vi "Shooter logic.vi"(0 "Low Pressure?":bool, 1 "Fire Main":bool, 2 "Fire 3":bool, 3 "Fire 2":bool, 4 "Change Arm State":bool, 5 "Grabber Override":bool, 6 "Release to Retract":u32=750, 7 "Grabber Button":bool, 8 "Time Between Open and Shoot":u32=250) -> ()   [LabVIEW 2013]
uses:
  <vilib>/Rock Robotics/WPI/Solenoid/WPI_SolenoidValue.ctl
  <vilib>/Rock Robotics/WPI/Solenoid/WPI_SolenoidSetEnum.vi
  <vilib>/addons/control/pid/pid.llb/PID (DBL).vi
  Robot Global Data.vi
  <vilib>/addons/control/pid/NI_PID_pid.lvlib
panel:
  in  "Up Position":dbl format="%.2f"
  in  "Arms IN/OUT":enum16{"Out", "In"}(ring)
  in  "Grabber Override State":enum16{"Sensors", "Buttons"}(ring)
  in  "Grab Sweet Spot inches fron sensor":dbl
  out "PID reinitalize?":bool
  in  "Down Position":dbl format="%.2f"
  in  "PID gains":T1={"proportional gain (Kc)"=1.0, "integral time (Ti, min)"=0.01, "derivative time (Td, min)"=0.0} {"derivative time (Td, min)" format="%.3f"; "integral time (Ti, min)" format="%.3f"; "proportional gain (Kc)" format="%.3f"}
  out "Arms Position":T2
  in  "Grabber State":enum16{"Up", "Going Down", "Down", "Going Up"}(ring)
  out "Shooter Position":T2
  in  "Launcher State":T3(ring)
  out "Tick":u32
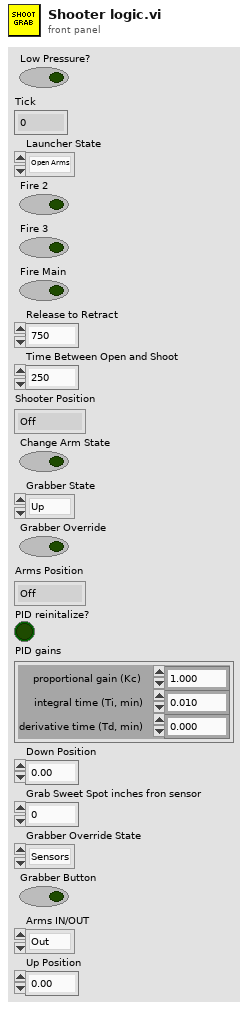
[diagram p1: front panel]
types:
  T1 = cluster{"proportional gain (Kc)":dbl, "integral time (Ti, min)":dbl, "derivative time (Td, min)":dbl}
  T2 = typedef "WPI_SolenoidValue.ctl" = enum16{"Off", "On", "Forward", "Reverse"}
  T3 = enum16{"Open Arms", "Arms Open", "Shoot", "Out", "Retract"}
  T4 = typedef "WPI_SolenoidDevRef.ctl" = cluster{"DevStatus":errorcluster, "Solenoid Module":T5, "Forward Solenoid Channel":T6, "Reverse Solenoid Channel":T6}
  T5 = typedef "FPGA_TypedefSolenoidModule.ctl" = enum16{"Solenoid Module 1", "Solenoid Module 2"}
  T6 = typedef "WPI_SolenoidChannel.ctl" = enum8{"Solenoid 1", "Solenoid 2", "Solenoid 3", "Solenoid 4", "Solenoid 5", "Solenoid 6", "Solenoid 7", "Solenoid 8", "Invalid"}
  T7 = typedef "WPI_DigitalInputDevRef.ctl" = cluster{"DevStatus":errorcluster, "DIO Channel":T8, "Digital Module":T9}
  T8 = typedef "FPGA_DIOChannel.ctl" = enum8{"DIO 1", "DIO 2", "DIO 3", "DIO 4", "DIO 5", "DIO 6", "DIO 7", "DIO 8", "DIO 9", "DIO 10", "DIO 11", "DIO 12", "DIO 13", "DIO 14", "Invalid"}
  T9 = typedef "FPGA_TypedefDigitalModule.ctl" = enum16{"Digital Module 1", "Digital Module 2"}
  T10 = typedef "WPI_AnalogChannelDevRef.ctl" = cluster{"DevStatus":errorcluster, "Analog Module":T11, "Analog Channel":T12}
  T11 = typedef "FPGA_TypedefAnalogModule.ctl" = enum16{"Analog Module 1", "Analog Module 2"}
  T12 = typedef "FPGA_AIChannel.ctl" = enum8{"AI 1", "AI 2", "AI 3", "AI 4", "AI 5", "AI 6", "AI 7", "AI 8", "Invalid"}
  T13 = typedef "WPI_MotorControlDeviceRef.ctl" = cluster{"DeviceStatus":errorcluster, "Type":enum16{"PWM", "CAN"}, "PWM":cluster{"Digital Module":T9, "PWM Channel":T14, "DeadBand":T15}, "CAN":cluster{"Device Number":u8, "Control Mode":T16, "Semaphore":T17, "Max Vout":dbl}, "Invert":bool, "TransformRef":T18, "InvTransformRef":T18}
  T14 = typedef "FPGA_DIOPWMChannel.ctl" = enum8{"PWM 1", "PWM 2", "PWM 3", "PWM 4", "PWM 5", "PWM 6", "PWM 7", "PWM 8", "PWM 9", "PWM 10", "Invalid"}
  T15 = typedef "WPI_PWMDeadband.ctl" = cluster{"Name":string, "maxPositivePwm":i32, "minPositivePwm":i32, "centerPwm":i32, "maxNegativePwm":i32, "minNegativePwm":i32, "angularRange":u16}
  T16 = typedef "WPI_CANJaguar_ControlMode.ctl" = enum8{"Percent VBus", "Current", "Speed", "Position", "Voltage"}
  T17 = typedef "Semaphore RefNum" = refnum<k1>
  T18 = typedef "WPI_PWMTransform_ConPane.ctl" = refnum<vi>
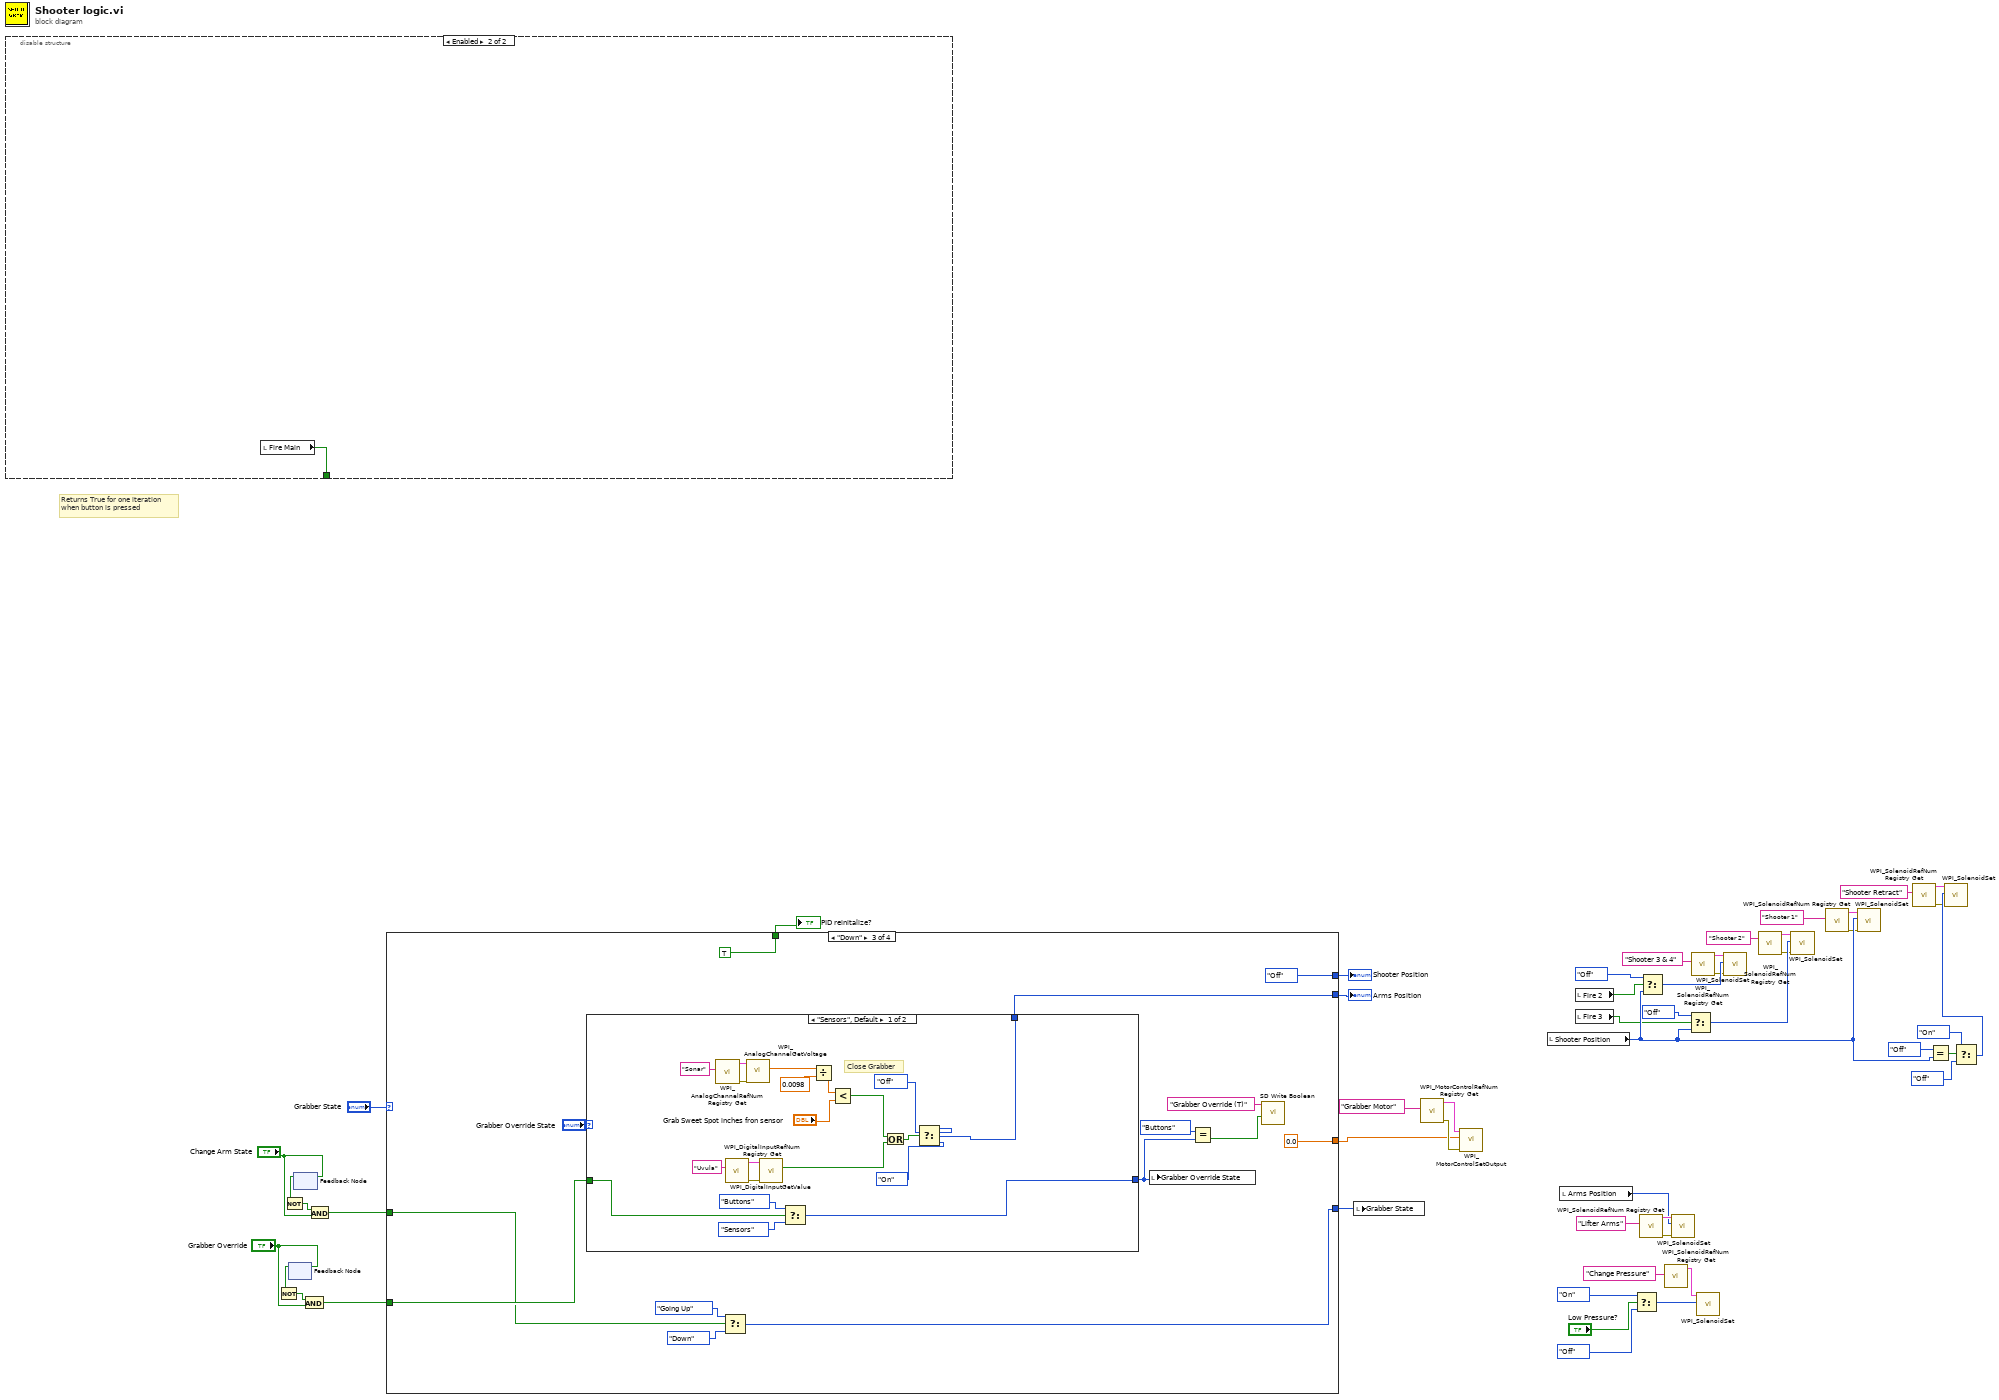
[diagram p0: block diagram]
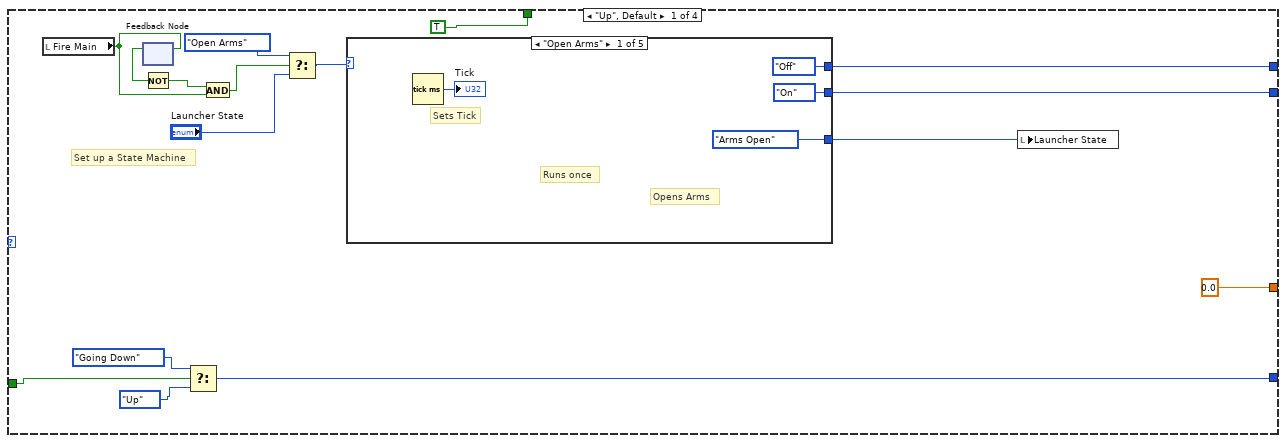
[diagram p2: hidden frame]
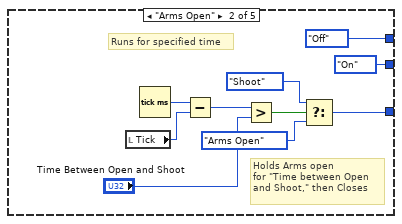
[diagram p3: hidden frame]
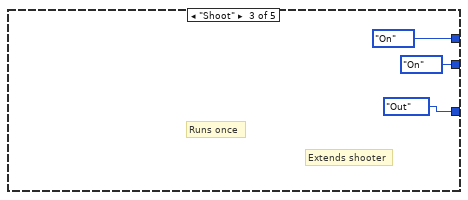
[diagram p4: hidden frame]
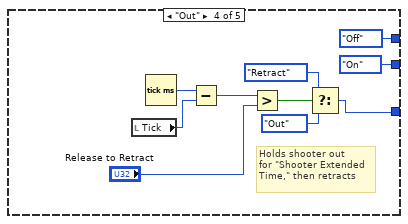
[diagram p5: hidden frame]
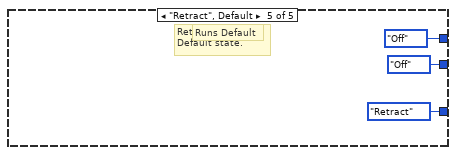
[diagram p6: hidden frame]
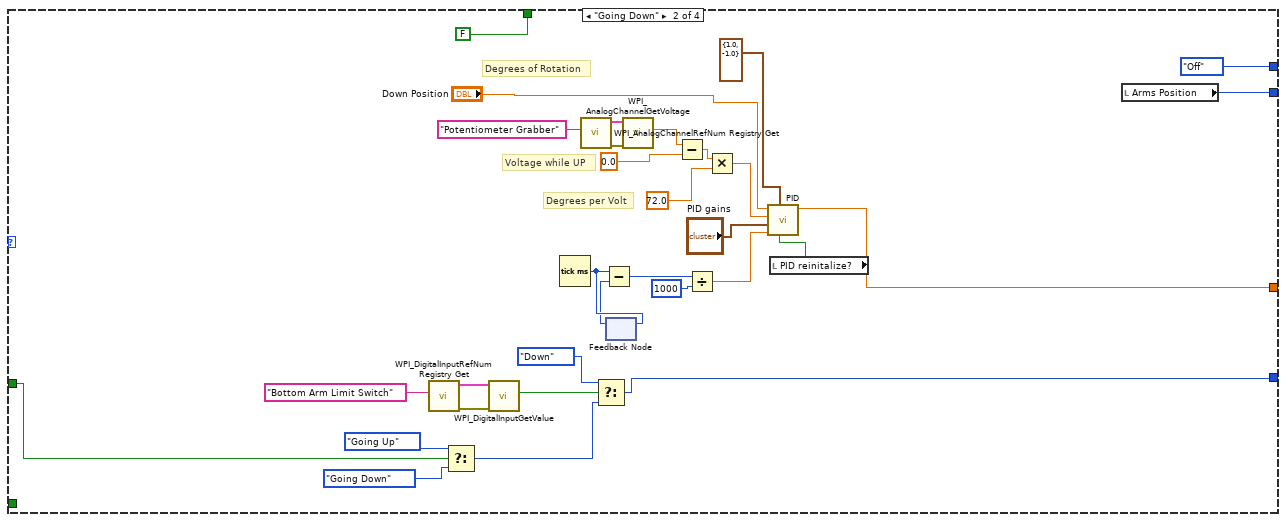
[diagram p7: hidden frame]
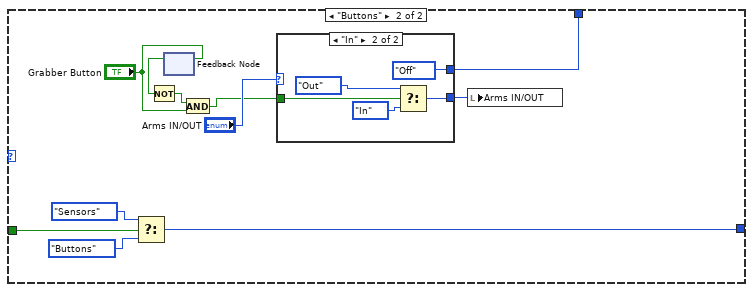
[diagram p8: hidden frame]
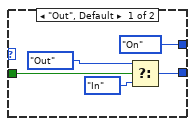
[diagram p9: hidden frame]
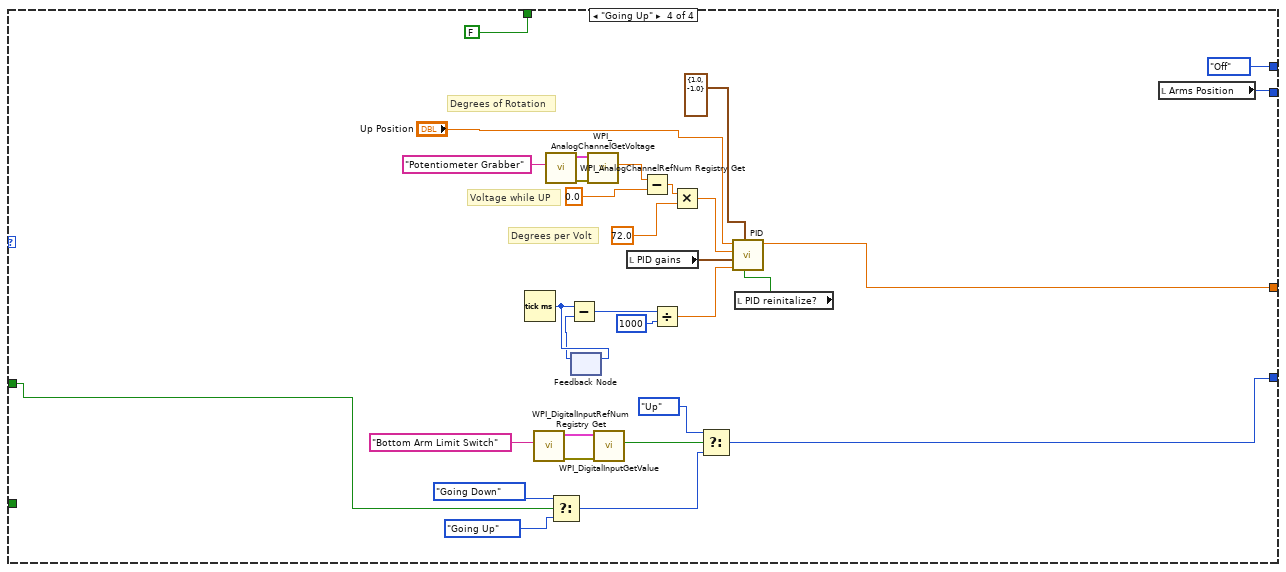
[diagram p10: hidden frame]
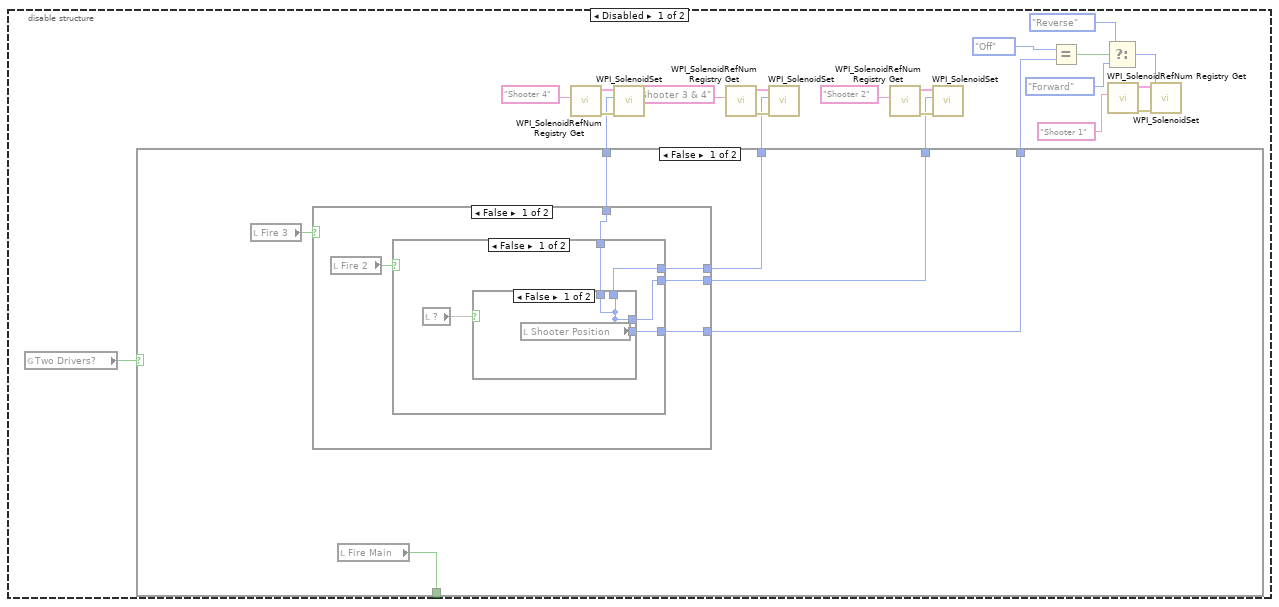
[diagram p11: hidden frame]
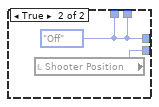
[diagram p12: hidden frame]
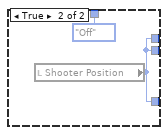
[diagram p13: hidden frame]
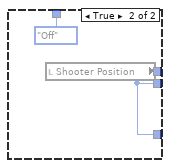
[diagram p14: hidden frame]
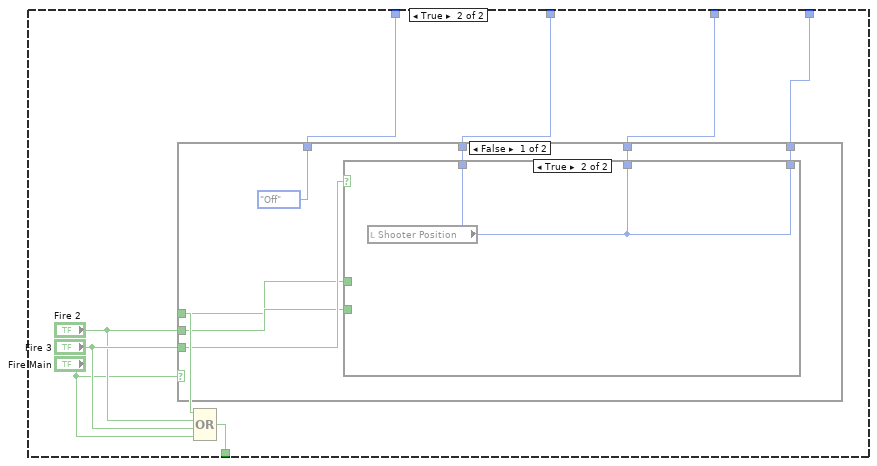
[diagram p15: hidden frame]
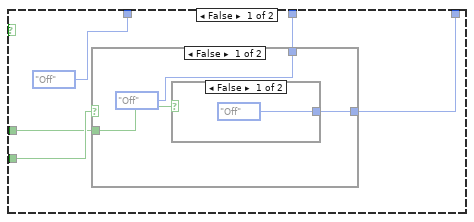
[diagram p16: hidden frame]
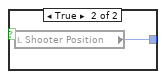
[diagram p17: hidden frame]
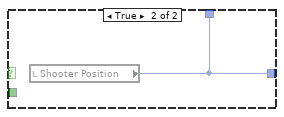
[diagram p18: hidden frame]
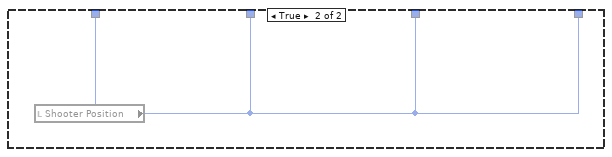
[diagram p19: hidden frame]
diagram:
  # "Returns True for one iteration\nwhen button is pressed"
  n1 = disable-structure shown="Enabled" {
    disable-tunnel: [w74 w127] -> _
    frame Disabled {
      n2 = global read "Robot Global Data.vi" "Two Drivers?"() -> (w73:bool)
      n3 = case shown="False" w73 {
        tunnel: [w80 w106] -> w74
        tunnel: [w75 w101] -> w55
        tunnel: [w78 w100] -> w54
        tunnel: [w77 w99] -> w53
        tunnel: [w76 w98] -> w52
        frame False {
          n4 = local read "Fire 3"() -> (w79:bool)
          n5 = case shown="False" w79 {
            tunnel: [w84 w97] -> w78
            tunnel: [w83 w97] -> w77
            tunnel: [w82 w97] -> w76
            tunnel: [w81 WPI_SolenoidValue."Off" ("Position")] -> w75
            frame False {
              n6 = local read "Fire 2"() -> (w85:bool)
              n7 = case shown="False" w85 {
                tunnel: [w87 w95] -> w84
                tunnel: [w88 w95] -> w83
                tunnel: [w89 w95] -> w82
                tunnel: [w86 WPI_SolenoidValue."Off" ("Position")] -> w81
                frame False {
                  n8 = local read item#-1() -> (w90)
                  n9 = case shown="False" w90 {
                    tunnel: [w91 w93] -> w89
                    tunnel: [w91 w92] -> w88
                    tunnel: [w91 w92] -> w87
                    tunnel: [w91 w92] -> w86
                    frame False {
                      n10 = local read "Shooter Position"() -> (w91:T2)
                    }
                    frame True {
                      w92 = WPI_SolenoidValue."Off" ("Position")
                      n11 = local read "Shooter Position"() -> (w93:T2)
                    }
                  }
                }
                frame True {
                  n12 = local read "Shooter Position"() -> (w95:T2)
                }
              }
            }
            frame True {
              n13 = local read "Shooter Position"() -> (w97:T2)
            }
          }
          n14 = local read "Fire Main"() -> (w80:bool)
        }
        frame True {
          n15 = Compound Arithmetic op=OR("Fire 2", "Fire 3", "Fire Main") -> (w106:bool, w103:bool)
          n16 = case shown="False" "Fire Main" {
            tunnel: [w109 w126] -> w98
            tunnel: [w110 w126] -> w99
            tunnel: [w111 w126] -> w100
            tunnel: [WPI_SolenoidValue."Off" ("Value") w126] -> w101
            tunnel: "Fire 3" -> [w112 _]
            tunnel: "Fire 2" -> [w108 _]
            tunnel: w103 -> [w107 _]
            frame False {
              n17 = case shown="True" w112 {
                tunnel: [WPI_SolenoidValue."Off" ("Value") w125] -> w111
                tunnel: [w118 w125] -> w110
                tunnel: [w117 w125] -> w109
                tunnel: w108 -> [w116 _]
                tunnel: w107 -> [w115 _]
                frame False {
                  n18 = case shown="False" w116 {
                    tunnel: [WPI_SolenoidValue."Off" ("Value") w124] -> w118
                    tunnel: [w119 w124] -> w117
                    tunnel: w115 -> [w120 _]
                    frame False {
                      n19 = case shown="False" w120 {
                        tunnel: [WPI_SolenoidValue."Off" ("Value") w123] -> w119
                        frame False {
                        }
                        frame True {
                          n20 = local read "Shooter Position"() -> (w123:T2)
                        }
                      }
                    }
                    frame True {
                      n21 = local read "Shooter Position"() -> (w124:T2)
                    }
                  }
                }
                frame True {
                  n22 = local read "Shooter Position"() -> (w125:T2)
                }
              }
            }
            frame True {
              n23 = local read "Shooter Position"() -> (w126:T2)
            }
          }
        }
      }
      n24 = call <vilib>:"WPI_SolenoidRefNum Registry Get.vi"("refnum name"="Shooter 4") -> ("error out"=w65:errorcluster, "SolenoidDevRef"=w66:T4)  [unwired: 9 in]
      n25 = call-poly <vilib>:"WPI_SolenoidSet.vi"("error in (no error)"=w65, "Value"=w55, "SolenoidDevRef"=w66) -> ()  [unwired: 7 in, 2 out]
      n26 = call <vilib>:"WPI_SolenoidRefNum Registry Get.vi"("refnum name"="Shooter 3 & 4") -> ("error out"=w68:errorcluster, "SolenoidDevRef"=w67:T4)  [unwired: 9 in]
      n27 = call-poly <vilib>:"WPI_SolenoidSet.vi"("error in (no error)"=w68, "Value"=w54, "SolenoidDevRef"=w67) -> ()  [unwired: 7 in, 2 out]
      n28 = call <vilib>:"WPI_SolenoidRefNum Registry Get.vi"("refnum name"="Shooter 2") -> ("error out"=w71:errorcluster, "SolenoidDevRef"=w72:T4)  [unwired: 9 in]
      n29 = call-poly <vilib>:"WPI_SolenoidSet.vi"("error in (no error)"=w71, "Value"=w53, "SolenoidDevRef"=w72) -> ()  [unwired: 7 in, 2 out]
      n30 = Equal?(x=WPI_SolenoidValue."Off" ("y"), y=w52) -> (x = y?=w58:bool)
      n31 = Select(t=WPI_SolenoidValue."Reverse" ("y"), s=w58, f=WPI_SolenoidValue."Forward" ("y")) -> (s? t:f=w61:T2)
      n32 = call <vilib>:"WPI_SolenoidRefNum Registry Get.vi"("refnum name"="Shooter 1") -> ("error out"=w57:errorcluster, "SolenoidDevRef"=w56:T4)  [unwired: 9 in]
      n33 = call-poly <vilib>:"WPI_SolenoidSet.vi"("error in (no error)"=w57, "Value"=w61, "SolenoidDevRef"=w56) -> ()  [unwired: 7 in, 2 out]
    }
    frame Enabled {
      n34 = local read "Fire Main"() -> (w127:bool)
    }
  }
  n35 = feedback #1() -> (w6:bool)  [unwired: 1 in]
  n36 = Not(x=w6) -> (.not. x?=w7:bool)
  n37 = feedback-in #1("Grabber Override") -> ()
  n38 = feedback-in #2("Change Arm State") -> ()
  n39 = feedback #2() -> (w46:bool)  [unwired: 1 in]
  n40 = Not(x=w46) -> (.not. x?=w45:bool)
  n41 = And(x=w7, y="Grabber Override") -> (x .and. y?=w4:bool)
  n42 = And(x=w45, y="Change Arm State") -> (x .and. y?=w44:bool)
  n43 = case shown="\"Down\"" "Grabber State" {
    tunnel: w44 -> [w132 w178 w208 w260]
    tunnel: [0.0 ("Output") w179 0.0 ("output") w271] -> w2
    tunnel: [w135 WPI_SolenoidValue."Off" ("Value") WPI_SolenoidValue."Off" ("Value") WPI_SolenoidValue."Off" ("Value")] -> w16
    tunnel: [w134 w204 w209 w288] -> w15
    tunnel: [w131 w197 w205 w261] -> w1
    tunnel: [TRUE FALSE TRUE FALSE] -> w8
    tunnel: w4 -> [_ _ w215 _]
    frame "Up", Default {
      # "Set up a State Machine"
      n44 = local read "Fire Main"() -> (w140:bool)
      n45 = feedback #3() -> (w141:bool)  [unwired: 1 in]
      n46 = feedback-in #3(w140) -> ()
      n47 = Not(x=w141) -> (.not. x?=w142:bool)
      n48 = Select(t=enum16{"Up", "Going Down", "Down", "Going Up"}."Going Down" ("Grabber State"), s=w132, f=enum16{"Up", "Going Down", "Down", "Going Up"}."Up" ("Grabber State")) -> (s? t:f=w131:enum16{"Up", "Going Down", "Down", "Going Up"})
      n49 = And(x=w142, y=w140) -> (x .and. y?=w137:bool)
      n50 = Select(t=T3."Open Arms", s=w137, f="Launcher State") -> (s? t:f=w139:T3)
      n51 = case shown="\"Open Arms\"" w139 {
        tunnel: [WPI_SolenoidValue."Off" ("Value") WPI_SolenoidValue."Off" ("Value") WPI_SolenoidValue."On" ("Value") WPI_SolenoidValue."Off" ("Value") WPI_SolenoidValue."Off" ("Value")] -> w135
        tunnel: [T3."Arms Open" ("Launcher State") w148 T3."Out" ("Launcher State") w163 T3."Retract" ("Launcher State")] -> w136
        tunnel: [WPI_SolenoidValue."On" ("Arm Position") WPI_SolenoidValue."On" ("Arm Position") WPI_SolenoidValue."On" ("Arm Position") WPI_SolenoidValue."On" ("Arm Position") WPI_SolenoidValue."Off" ("Arm Position")] -> w134
        frame "Open Arms" {
          # "Opens Arms"
          # "Runs once"
          # "Sets Tick"
          n52 = Tick Count (ms)() -> (millisecond timer value=→"Tick":u32)
        }
        frame "Arms Open" {
          # "Runs for specified time"
          # "Holds Arms open\nfor \"Time between Open\nand Shoot,\" then Closes"
          n53 = local read "Tick"() -> (w156:u32)
          n54 = Tick Count (ms)() -> (millisecond timer value=w157:u32)
          n55 = Subtract(x=w157, y=w156) -> (x-y=w155:u32)
          n56 = Greater?(x=w155, y="Time Between Open and Shoot") -> (0:w154:bool)
          n57 = Select(t=T3."Shoot" ("Launcher State"), s=w154, f=T3."Arms Open" ("Launcher State")) -> (s? t:f=w148:T3)
        }
        frame "Shoot" {
          # "Runs once"
          # "Extends shooter"
        }
        frame "Out" {
          # "Holds shooter out\nfor \"Shooter Extended\nTime,\" then retracts"
          n58 = local read "Tick"() -> (w169:u32)
          n59 = Tick Count (ms)() -> (millisecond timer value=w170:u32)
          n60 = Subtract(x=w170, y=w169) -> (x-y=w168:u32)
          n61 = Greater?(x=w168, y="Release to Retract") -> (0:w167:bool)
          n62 = Select(t=T3."Retract" ("Launcher State"), s=w167, f=T3."Out" ("Launcher State")) -> (s? t:f=w163:T3)
        }
        frame "Retract", Default {
          # "Runs Default"
          # "Retracts Shooter, \nDefault state."
        }
      }
      n63 = local write "Launcher State"(w136) -> ()
    }
    frame "Going Down" {
      # "Degrees of Rotation"
      # "Degrees per Volt"
      # "Voltage while UP"
      n64 = call <vilib>:"WPI_DigitalInputRefNum Registry Get.vi"("refnum name"="Bottom Arm Limit Switch") -> ("error out"=w201:errorcluster, "DigitalInputDevRef"=w200:T7)  [unwired: 9 in]
      n65 = Select(t=enum16{"Up", "Going Down", "Down", "Going Up"}."Going Up", s=w178, f=enum16{"Up", "Going Down", "Down", "Going Up"}."Going Down" ("Grabber State")) -> (s? t:f=w174:enum16{"Up", "Going Down", "Down", "Going Up"})
      n66 = call <vilib>:"WPI_DigitalInputGetValue.vi"("error in (no error)"=w201, "DigitalInputDevRef"=w200) -> ("Value"=w198:bool)  [unwired: 7 in, 2 out]
      n67 = Tick Count (ms)() -> (millisecond timer value=w181:u32)
      n68 = call <vilib>:"WPI_AnalogChannelRefNum Registry Get.vi"("refnum name"="Potentiometer Grabber") -> ("error out"=w185:errorcluster, "AIDeviceRef"=w184:T10)  [unwired: 9 in]
      n69 = Select(t=enum16{"Up", "Going Down", "Down", "Going Up"}."Down" ("Grabber State"), s=w198, f=w174) -> (s? t:f=w197:enum16{"Up", "Going Down", "Down", "Going Up"})
      n70 = feedback #4() -> (w180:u32)  [unwired: 1 in]
      n71 = Subtract(x=w181, y=w180) -> (x-y=w186:u32)
      n72 = feedback-in #4(w181) -> ()
      n73 = call <vilib>:"WPI_AnalogChannelGetVoltage.vi"("error in (no error)"=w185, "AIDeviceRef"=w184) -> ("Voltage"=w189:dbl)  [unwired: 7 in, 2 out]
      n74 = Subtract(x=w189, y=0.0) -> (x-y=w191:dbl)
      n75 = Divide(x=w186, y=u32 1000) -> (x/y=w188:dbl)
      n76 = Multiply(x=w191, y=72.0) -> (x*y=w193:dbl)
      n77 = local read "PID reinitalize?"() -> (w195:bool)
      n78 = call-poly <vilib>:"PID.vi"("reinitialize? (F)"=w195, "output range"=cluster{"output high":dbl, "output low":dbl} {"output high"=1.0, "output low"=-1.0}, "dt (s)"=w188, "PID gains"="PID gains", "process variable"=w193, "setpoint"="Down Position") -> ("output"=w179:dbl)  [unwired: 4 in, 1 out]
      n79 = local read "Arms Position"() -> (w204:T2)
    }
    frame "Down" {
      n80 = case shown="\"Sensors\", Default" "Grabber Override State" {
        tunnel: w215 -> [w228 w249]
        tunnel: [w226 w246] -> w212
        tunnel: [w225 w239] -> w209
        frame "Sensors", Default {
          # "Close Grabber"
          n81 = call <vilib>:"WPI_AnalogChannelRefNum Registry Get.vi"("refnum name"="Sonar") -> ("error out"=w224:errorcluster, "AIDeviceRef"=w223:T10)  [unwired: 9 in]
          n82 = call <vilib>:"WPI_DigitalInputRefNum Registry Get.vi"("refnum name"="Uvula") -> ("error out"=w236:errorcluster, "DigitalInputDevRef"=w235:T7)  [unwired: 9 in]
          n83 = call <vilib>:"WPI_AnalogChannelGetVoltage.vi"("error in (no error)"=w224, "AIDeviceRef"=w223) -> ("Voltage"=w221:dbl)  [unwired: 7 in, 2 out]
          n84 = call <vilib>:"WPI_DigitalInputGetValue.vi"("error in (no error)"=w236, "DigitalInputDevRef"=w235) -> ("Value"=w233:bool)  [unwired: 7 in, 2 out]
          n85 = Select(t=enum16{"Sensors", "Buttons"}."Buttons", s=w228, f=enum16{"Sensors", "Buttons"}."Sensors") -> (s? t:f=w226:enum16{"Sensors", "Buttons"})
          n86 = Divide(x=w221, y=0.0098) -> (x/y=w222:dbl)
          n87 = Less?(x=w222, y="Grab Sweet Spot inches fron sensor") -> (x < y?=w234:bool)
          n88 = Or(x=w234, y=w233) -> (x .or. y?=w232:bool)
          n89 = Select(t=WPI_SolenoidValue."Off" ("Arms Position"), s=w232, f=WPI_SolenoidValue."On") -> (s? t:f=w225:T2)
        }
        frame "Buttons" {
          n90 = Select(t=enum16{"Sensors", "Buttons"}."Sensors", s=w249, f=enum16{"Sensors", "Buttons"}."Buttons") -> (s? t:f=w246:enum16{"Sensors", "Buttons"})
          n91 = feedback #5() -> (w245:bool)  [unwired: 1 in]
          n92 = Not(x=w245) -> (.not. x?=w244:bool)
          n93 = feedback-in #5("Grabber Button") -> ()
          n94 = And(x=w244, y="Grabber Button") -> (x .and. y?=w241:bool)
          n95 = case shown="\"In\"" "Arms IN/OUT" {
            tunnel: w241 -> [w252 w258]
            tunnel: [w251 w256] -> w240
            tunnel: [WPI_SolenoidValue."On" ("f") WPI_SolenoidValue."Off" ("f")] -> w239
            frame "Out", Default {
              n96 = Select(t=enum16{"Out", "In"}."Out" ("Arms IN/OUT"), s=w252, f=enum16{"Out", "In"}."In") -> (s? t:f=w251:enum16{"Out", "In"})
            }
            frame "In" {
              n97 = Select(t=enum16{"Out", "In"}."Out" ("Arms IN/OUT"), s=w258, f=enum16{"Out", "In"}."In") -> (s? t:f=w256:enum16{"Out", "In"})
            }
          }
          n98 = local write "Arms IN/OUT"(w240) -> ()
        }
      }
      n99 = Select(t=enum16{"Up", "Going Down", "Down", "Going Up"}."Going Up" ("Grabber State"), s=w208, f=enum16{"Up", "Going Down", "Down", "Going Up"}."Down" ("Grabber State")) -> (s? t:f=w205:enum16{"Up", "Going Down", "Down", "Going Up"})
      n100 = local write "Grabber Override State"(w212) -> ()
      n101 = Equal?(x=enum16{"Sensors", "Buttons"}."Buttons", y=w212) -> (x = y?=w210:bool)
      n102 = call <vilib>:"SD Write Boolean.vi"("Boolean"=w210, "Name"="Grabber Override (T)") -> ()  [unwired: 8 in, 2 out]
    }
    frame "Going Up" {
      # "Degrees of Rotation"
      # "Degrees per Volt"
      # "Voltage while UP"
      n103 = Tick Count (ms)() -> (millisecond timer value=w273:u32)
      n104 = call <vilib>:"WPI_DigitalInputRefNum Registry Get.vi"("refnum name"="Bottom Arm Limit Switch") -> ("error out"=w269:errorcluster, "DigitalInputDevRef"=w268:T7)  [unwired: 9 in]
      n105 = call <vilib>:"WPI_AnalogChannelRefNum Registry Get.vi"("refnum name"="Potentiometer Grabber") -> ("error out"=w285:errorcluster, "AIDeviceRef"=w286:T10)  [unwired: 9 in]
      n106 = Select(t=enum16{"Up", "Going Down", "Down", "Going Up"}."Going Down", s=w260, f=enum16{"Up", "Going Down", "Down", "Going Up"}."Going Up" ("Grabber State")) -> (s? t:f=w262:enum16{"Up", "Going Down", "Down", "Going Up"})
      n107 = feedback #6() -> (w272:u32)  [unwired: 1 in]
      n108 = Subtract(x=w273, y=w272) -> (x-y=w284:u32)
      n109 = feedback-in #6(w273) -> ()
      n110 = call <vilib>:"WPI_AnalogChannelGetVoltage.vi"("error in (no error)"=w285, "AIDeviceRef"=w286) -> ("Voltage"=w281:dbl)  [unwired: 7 in, 2 out]
      n111 = call <vilib>:"WPI_DigitalInputGetValue.vi"("error in (no error)"=w269, "DigitalInputDevRef"=w268) -> ("Value"=w266:bool)  [unwired: 7 in, 2 out]
      n112 = local read "PID gains"() -> (w270:T1)
      n113 = Subtract(x=w281, y=0.0) -> (x-y=w279:dbl)
      n114 = Divide(x=w284, y=u32 1000) -> (x/y=w282:dbl)
      n115 = Multiply(x=w279, y=72.0) -> (x*y=w277:dbl)
      n116 = Select(t=enum16{"Up", "Going Down", "Down", "Going Up"}."Up" ("Grabber State"), s=w266, f=w262) -> (s? t:f=w261:enum16{"Up", "Going Down", "Down", "Going Up"})
      n117 = local read "PID reinitalize?"() -> (w275:bool)
      n118 = call-poly <vilib>:"PID.vi"("reinitialize? (F)"=w275, "output range"=cluster{"output high":dbl, "output low":dbl} {"output high"=1.0, "output low"=-1.0}, "dt (s)"=w282, "PID gains"=w270, "process variable"=w277, "setpoint"="Up Position") -> ("output"=w271:dbl)  [unwired: 4 in, 1 out]
      n119 = local read "Arms Position"() -> (w288:T2)
    }
  }
  "Shooter Position" <- w16
  "Arms Position" <- w15
  "PID reinitalize?" <- w8
  n120 = local write "Grabber State"(w1) -> ()
  n121 = call <vilib>:"WPI_MotorControlRefNum Registry Get.vi"("refnum name"="Grabber Motor") -> ("error out"=w51:errorcluster, "MotorControlDevRef"=w50:T13)  [unwired: 9 in]
  n122 = call <vilib>:"WPI_MotorControlSetOutput.vi"("error in (no error)"=w51, "Output"=w2, "MotorControlDevRef"=w50) -> ()  [unwired: 6 in, 3 out]
  n123 = local read "Shooter Position"() -> (w36:T2)
  n124 = local read "Arms Position"() -> (w3:T2)
  n125 = local read "Fire 2"() -> (w30:bool)
  n126 = local read "Fire 3"() -> (w26:bool)
  n127 = Select(t=WPI_SolenoidValue."On", s="Low Pressure?", f=WPI_SolenoidValue."Off" ("t")) -> (s? t:f=w10:T2)
  n128 = call <vilib>:"WPI_SolenoidRefNum Registry Get.vi"("refnum name"="Lifter Arms") -> ("error out"=w42:errorcluster, "SolenoidDevRef"=w41:T4)  [unwired: 9 in]
  n129 = Select(t=WPI_SolenoidValue."Off", s=w30, f=w36) -> (s? t:f=w31:T2)
  n130 = call <vilib>:"WPI_SolenoidRefNum Registry Get.vi"("refnum name"="Change Pressure") -> ("SolenoidDevRef"=w14:T4)  [unwired: 9 in, 1 out]
  n131 = call-poly <vilib>:"WPI_SolenoidSet.vi"("error in (no error)"=w42, "Value"=w3, "SolenoidDevRef"=w41) -> ()  [unwired: 7 in, 2 out]
  n132 = Select(t=WPI_SolenoidValue."Off", s=w26, f=w36) -> (s? t:f=w27:T2)
  n133 = call <vilib>:"WPI_SolenoidRefNum Registry Get.vi"("refnum name"="Shooter 3 & 4") -> ("error out"=w21:errorcluster, "SolenoidDevRef"=w22:T4)  [unwired: 9 in]
  n134 = call-poly <vilib>:"WPI_SolenoidSet.vi"("Value"=w10, "SolenoidDevRef"=w14) -> ()  [unwired: 8 in, 2 out]
  n135 = call-poly <vilib>:"WPI_SolenoidSet.vi"("error in (no error)"=w21, "Value"=w31, "SolenoidDevRef"=w22) -> ()  [unwired: 7 in, 2 out]
  n136 = call <vilib>:"WPI_SolenoidRefNum Registry Get.vi"("refnum name"="Shooter 2") -> ("error out"=w18:errorcluster, "SolenoidDevRef"=w17:T4)  [unwired: 9 in]
  n137 = call-poly <vilib>:"WPI_SolenoidSet.vi"("error in (no error)"=w18, "Value"=w27, "SolenoidDevRef"=w17) -> ()  [unwired: 7 in, 2 out]
  n138 = call <vilib>:"WPI_SolenoidRefNum Registry Get.vi"("refnum name"="Shooter 1") -> ("error out"=w24:errorcluster, "SolenoidDevRef"=w25:T4)  [unwired: 9 in]
  n139 = call-poly <vilib>:"WPI_SolenoidSet.vi"("error in (no error)"=w24, "Value"=w36, "SolenoidDevRef"=w25) -> ()  [unwired: 7 in, 2 out]
  n140 = call <vilib>:"WPI_SolenoidRefNum Registry Get.vi"("refnum name"="Shooter Retract") -> ("error out"=w33:errorcluster, "SolenoidDevRef"=w32:T4)  [unwired: 9 in]
  n141 = Equal?(x=WPI_SolenoidValue."Off", y=w36) -> (x = y?=w35:bool)
  n142 = Select(t=WPI_SolenoidValue."On" ("x"), s=w35, f=WPI_SolenoidValue."Off" ("x")) -> (s? t:f=w40:T2)
  n143 = call-poly <vilib>:"WPI_SolenoidSet.vi"("error in (no error)"=w33, "Value"=w40, "SolenoidDevRef"=w32) -> ()  [unwired: 7 in, 2 out]
